vi "Sensor_Read.vi"(4 "error in (no error)":errorcluster, 5 "write ED33":string="?\\r", 6 "Clear":bool, 7 "Sensor Box":string(combo), 8 "Port Sensors":refnum<visa-resource-name>="COM6", 9 "Sensors Active?":bool, 10 "ED33 Active?":bool, 11 "Port ED33":refnum<visa-resource-name>="COM7") -> (2 "Sensors_output":string[][](array[string]), 3 "ED33_output":string[][](array[string]))   [LabVIEW 2013]
uses:
  <vilib>/Instr/_visa.llb/VISA Configure Serial Port (Instr).vi
panel:
  out "read Sensors":string
  out "read ED33":string
  out "error out 2":errorcluster
  out "error out":errorcluster
  out "Bytes at Serial Port 2":u32
  in  "timeout (10sec) 2":u32=10000
  in  "flow control (0:none) 2":u16(ring) items=["None", "XON/XOFF", "RTS/CTS", "XON/XOFF & RTS/CTS", "DTR/DSR", "XON/XOFF & DTR/DSR"]
  in  "stop bits (10: 1 bit) 2":u16(ring)=10 items=["1.0"=10, "1.5"=15, "2.0"=20]
  in  "parity (0:none) 2":enum16{"None", "Odd", "Even", "Mark", "Space"}(ring)
  in  "data bits (8) 2":u16=8
  in  "baud rate (ED33)":u32=115200
  out "Bytes at Serial Port":u32
  in  "write Sensors":string="raw_all"
  in  "timeout (10sec)":u32=10000
  in  "flow control (0:none)":u16(ring) items=["None", "XON/XOFF", "RTS/CTS", "XON/XOFF & RTS/CTS", "DTR/DSR", "XON/XOFF & DTR/DSR"]
  in  "stop bits (10: 1 bit)":u16(ring)=10 items=["1.0"=10, "1.5"=15, "2.0"=20]
  in  "parity (0:none)":enum16{"None", "Odd", "Even", "Mark", "Space"}(ring)
  in  "data bits (8)":u16=8
  in  "baud rate (Sensors)":u32=115200
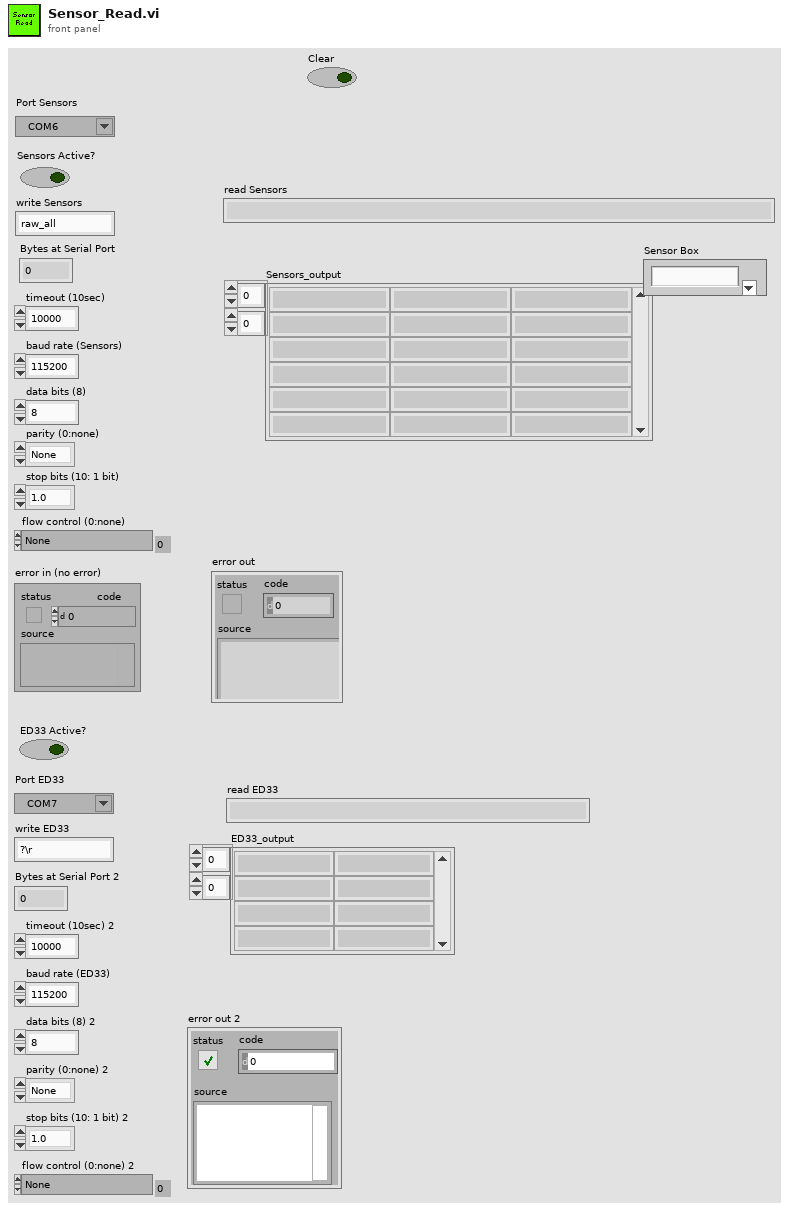
[diagram p1: front panel]
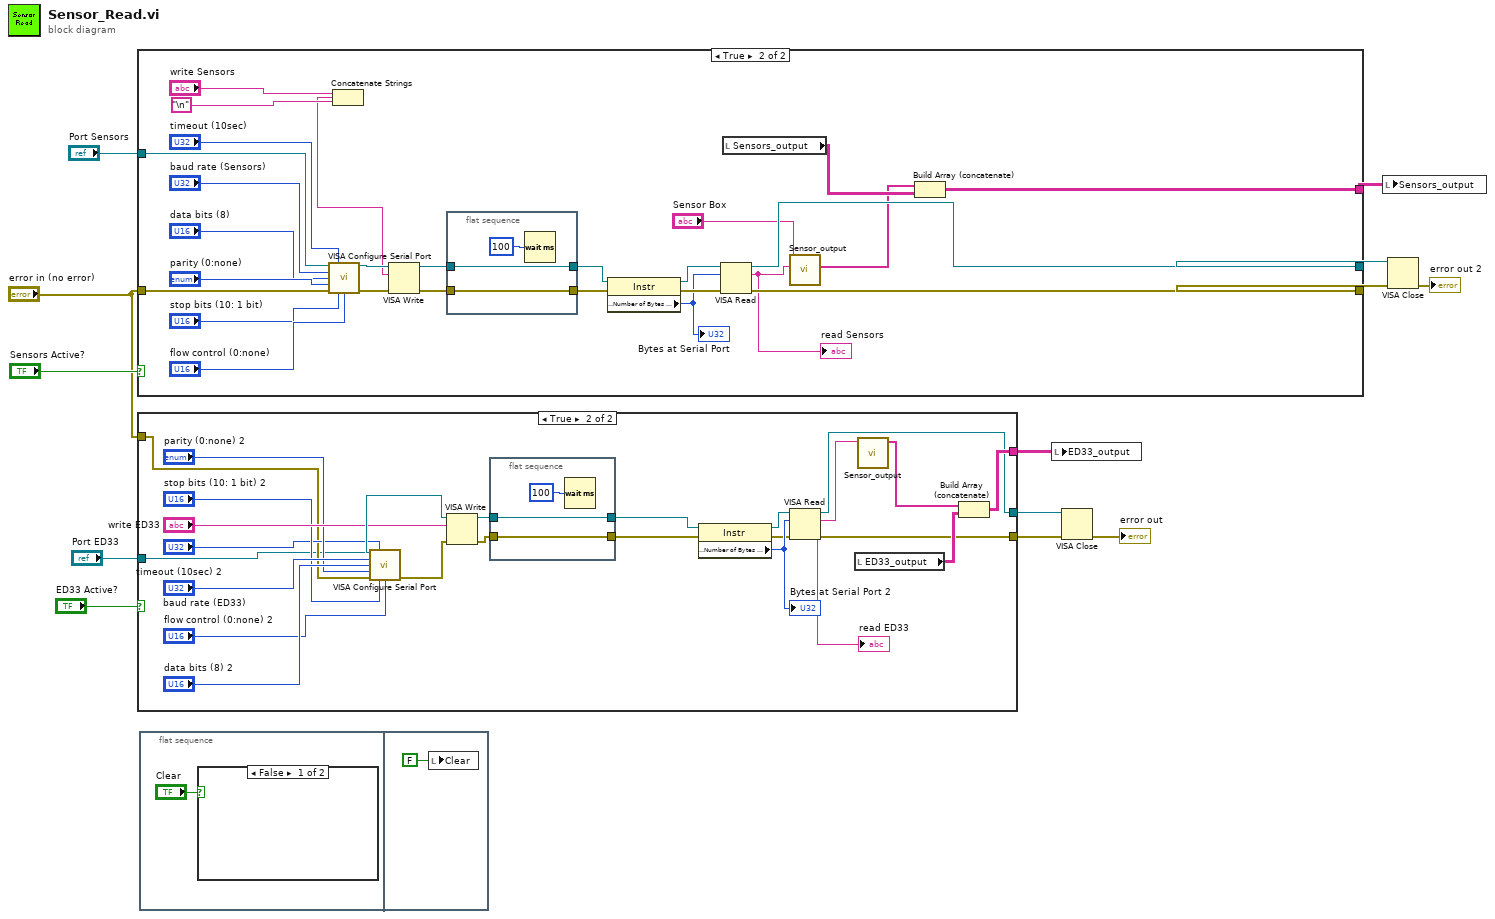
[diagram p0: block diagram]
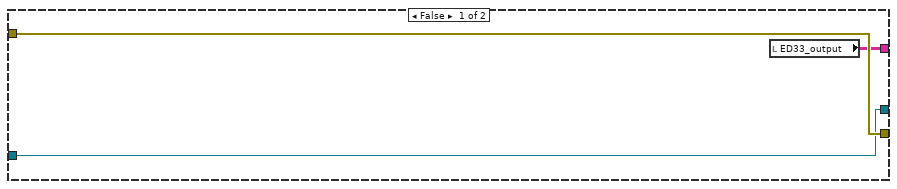
[diagram p2: hidden frame]
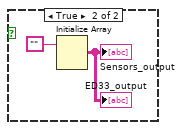
[diagram p3: hidden frame]
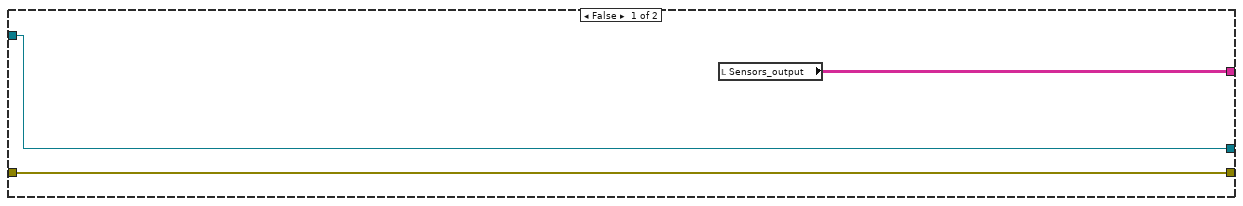
[diagram p4: hidden frame]
diagram:
  n1 = case shown="True" "Sensors Active?" {
    tunnel: "Port Sensors" -> [w16 w37]
    tunnel: "error in (no error)" -> [w15 w36]
    tunnel: [w16 w26] -> w6
    tunnel: [w15 w25] -> w5
    tunnel: [w14 w24] -> w2
    frame False {
      n2 = local read "Sensors_output"() -> (w14:string[][])
    }
    frame True {
      n3 = call-poly "VISA Configure Serial Port"("VISA resource name"=w37, "timeout (10sec)"="timeout (10sec)", "baud rate (9600)"="baud rate (Sensors)", "data bits (8)"="data bits (8)", "parity (0:none)"="parity (0:none)", "error in (no error)"=w36, "stop bits (10: 1 bit)"="stop bits (10: 1 bit)", "flow control (0:none)"="flow control (0:none)") -> ("VISA resource name out"=w28:refnum<visa-resource-name>, "error out"=w27:errorcluster)  [unwired: 1 in, 5 out]
      n4 = Concatenate Strings("write Sensors", "\n") -> (w17:string)
      n5 = VISA Write(VISA resource name=w28, write buffer=w17, error in (no error)=w27) -> (VISA resource name out=w29:refnum<visa-resource-name>, error out=w32:errorcluster)  [unwired: 1 out]
      n6 = flat-sequence {
        tunnel: w29 -> [w45]
        tunnel: [w45] -> w30
        tunnel: [w44] -> w31
        tunnel: w32 -> [w44]
        frame #0 {
          n7 = Wait (ms)(milliseconds to wait=u32 100) -> ()  [unwired: 1 out]
        }
      }
      n8 = property class="Instr"(reference=w30, error in=w31) -> (reference out=w35:refnum<visa-resource-name>, error out=w34:errorcluster, "Serial Settings:Number of Bytes at Serial Port"=w33:u32)
      "Bytes at Serial Port" <- w33
      n9 = VISA Read(VISA resource name=w35, byte count=w33, error in (no error)=w34) -> (VISA resource name out=w26:refnum<visa-resource-name>, read buffer=w23:string, error out=w25:errorcluster)  [unwired: 1 out]
      "read Sensors" <- w23
      n10 = local read "Sensors_output"() -> (w22:string[][])
      n11 = call "Sensor_output.vi"("Sensor Box"="Sensor Box", "Sensors"=w23) -> ("Sensors_output"=w21:string[])  [unwired: 5 in, 1 out]
      n12 = Build Array (concatenate)(w21, w22) -> (w24:string[][])
    }
  }
  n13 = case shown="True" "ED33 Active?" {
    tunnel: [w47 w55] -> w3
    tunnel: [w48 w54] -> w9
    tunnel: [w49 w53] -> w11
    tunnel: "error in (no error)" -> [w49 w52]
    tunnel: "Port ED33" -> [w48 w51]
    frame False {
      n14 = local read "ED33_output"() -> (w47:string[][])
    }
    frame True {
      n15 = call-poly "VISA Configure Serial Port"("VISA resource name"=w51, "timeout (10sec)"="timeout (10sec) 2", "baud rate (9600)"="baud rate (ED33)", "data bits (8)"="data bits (8) 2", "parity (0:none)"="parity (0:none) 2", "error in (no error)"=w52, "stop bits (10: 1 bit)"="stop bits (10: 1 bit) 2", "flow control (0:none)"="flow control (0:none) 2") -> ("VISA resource name out"=w72:refnum<visa-resource-name>, "error out"=w71:errorcluster)  [unwired: 1 in, 5 out]
      n16 = VISA Write(VISA resource name=w72, write buffer="write ED33", error in (no error)=w71) -> (VISA resource name out=w69:refnum<visa-resource-name>, error out=w66:errorcluster)  [unwired: 1 out]
      n17 = flat-sequence {
        tunnel: w69 -> [w75]
        tunnel: [w75] -> w68
        tunnel: [w74] -> w67
        tunnel: w66 -> [w74]
        frame #0 {
          n18 = Wait (ms)(milliseconds to wait=u32 100) -> ()  [unwired: 1 out]
        }
      }
      n19 = property class="Instr"(reference=w68, error in=w67) -> (reference out=w63:refnum<visa-resource-name>, error out=w64:errorcluster, "Serial Settings:Number of Bytes at Serial Port"=w65:u32)
      "Bytes at Serial Port 2" <- w65
      n20 = VISA Read(VISA resource name=w63, byte count=w65, error in (no error)=w64) -> (VISA resource name out=w54:refnum<visa-resource-name>, read buffer=w62:string, error out=w53:errorcluster)  [unwired: 1 out]
      "read ED33" <- w62
      n21 = local read "ED33_output"() -> (w73:string[][])
      n22 = call "Sensor_output.vi"("ED33"=w62) -> ("ED33_output"=w50:string[])  [unwired: 6 in, 1 out]
      n23 = Build Array (concatenate)(w50, w73) -> (w55:string[][])
    }
  }
  n24 = flat-sequence {
    frame #0 {
      n25 = case shown="False" "Clear" {
        frame False {
        }
        frame True {
          n26 = Initialize Array("") -> (→"Sensors_output" →"ED33_output":string[][])  [unwired: 2 in]
        }
      }
    }
    frame #1 {
      n27 = local write "Clear"(FALSE ("Clear")) -> ()
    }
  }
  n28 = local write "ED33_output"(w3) -> ()
  n29 = VISA Close(VISA resource name=w9, error in (no error)=w11) -> (error out=→"error out":errorcluster)
  n30 = local write "Sensors_output"(w2) -> ()
  n31 = VISA Close(VISA resource name=w6, error in (no error)=w5) -> (error out=→"error out 2":errorcluster)
